vi "PWM FPGA.vi"(7 "引用句柄输入":refnum<k21>, 11 "PWM FT":u32) -> ()   [LabVIEW 2017]
uses:
  <vilib>/rvi/eio/common/nirviEmuTemplateMethod_errors.vi
  <vilib>/eio/EIONode/EIONode.xnode
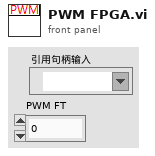
[diagram p1: front panel]
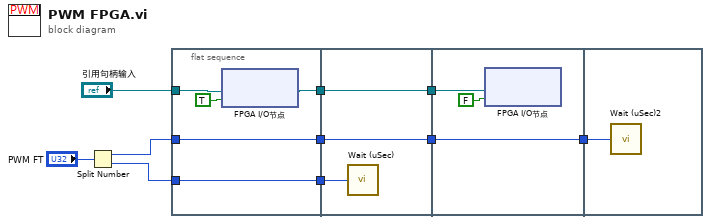
[diagram p0: block diagram]
diagram:
  n1 = Split Number(x="PWM FT") -> (hi(x)=w3:u16, lo(x)=w2:u16)
  n2 = flat-sequence {
    tunnel: "引用句柄输入" -> [w15]
    tunnel: [w14] -> w10
    tunnel: w2 -> [w13]
    tunnel: [w13] -> w9
    tunnel: w3 -> [w12]
    tunnel: [w12] -> w8
    tunnel: w10 -> [w18]
    tunnel: w9 -> [w17]
    tunnel: [w18] -> w7
    tunnel: w8 -> [w16]
    tunnel: [w16] -> w6
    tunnel: w7 -> [w21]
    tunnel: w6 -> [w20]
    tunnel: [w20] -> w5
    tunnel: w5 -> [w22]
    frame #0 {
      n3 = xnode "FPGA I/O节点"("I/O项"=TRUE ("invert pulse (F)"), "FPGA I/O输入"=w15) -> ("FPGA I/O输出"=w14:refnum<k21>)
    }
    frame #1 {
      n4 = call "Wait (uSec)"("Count(uSec)"=w17) -> ()  [unwired: 1 out]
    }
    frame #2 {
      n5 = xnode "FPGA I/O节点"("I/O项"=FALSE ("invert pulse (F)"), "FPGA I/O输入"=w21) -> ()  [unwired: 1 out]
    }
    frame #3 {
      n6 = call "Wait (uSec)2"("Count(uSec)"=w22) -> ()  [unwired: 1 out]
    }
  }
